vi "Write Registers.vi"(8 "error in (no error)":errorcluster, 9 "registers":u16[](array[numeric]), 10 "address":i32, 11 "modbus in":refnum<class "libmodbus.lvclass">) -> (0 "error out":errorcluster, 3 "modbus out":refnum<class "libmodbus.lvclass">)   [LabVIEW 2017, in "libmodbus.lvlib" / "libmodbus.lvclass"]
doc: "Writes many modbus holding registers."
uses:
  libmodbus.lvclass
  libmodbus.lvclass/libmodbus.ctl
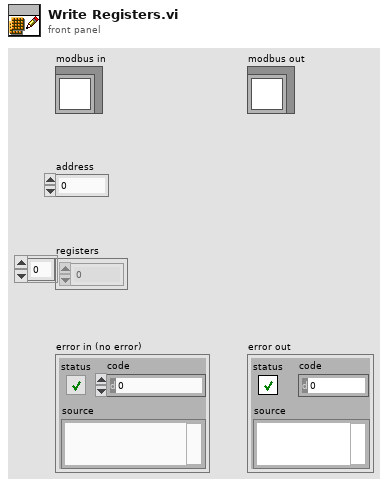
[diagram p1: front panel]
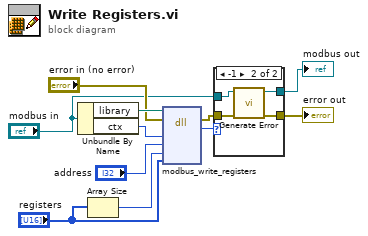
[diagram p0: block diagram]
diagram:
  n1 = Unbundle By Name("modbus in") -> ("library"=w10:path, "ctx"=w11:i64)
  n2 = Array Size(array="registers") -> (size(s)=w1:i32)
  n3 = dll-call lib="?" fn="modbus_write_registers"(path in=w10, error in="error in (no error)", "ctx"=w11, "addr"="address", "nb"=w1, "src"="registers") -> (error out=w6:errorcluster, "int"=w8:i32)  [unwired: 5 in, 1 out]
  n4 = case shown="-1" w8 {
    tunnel: [w13 w16] -> w7
    tunnel: w6 -> [w13 w17]
    tunnel: "modbus in" -> [w12 w15]
    tunnel: [w12 w14] -> w4
    frame Default {
    }
    frame -1 {
      n5 = call "Generate Error.vi"("error in (no error)"=w17, "modbus in"=w15) -> ("error out"=w16:errorcluster, "modbus out"=w14:refnum<class "libmodbus.lvclass">)  [unwired: 8 in]
    }
  }
  "modbus out" <- w4
  "error out" <- w7
